vi "MGI Linear Fit.vi"(9 "Weights (equal)[]":dbl[](array[numeric]) format="%#.6g", 10 "Xin[]":dbl[](array[numeric]) format="%#.6g", 11 "Yin[]":dbl[](array[numeric]) format="%#.6g") -> (0 "Intercept":dbl, 1 "Slope":dbl, 2 "Xout[]":dbl[](array[numeric]), 3 "Yout[]":dbl[](array[numeric]))   [LabVIEW 2020]
doc: "Finds the least squares linear fit parameters for the provided data. If the range of x values is not greater than the range of y values, then the fit is performed with the x and y values reversed, with the outputs converted back to the original orientation. If the optional Weights input is empty or unwired, then the weights used in the fit are all set to 1 (equal weighting).\n\nAuthored by David A Moore\nsupport@mooregoodideas.com\nwww.mooregoodideas.com\n\nCopyright (c) 2010, Moore Good Ideas, Inc.\n\nAll rights reserved.\n\nRedistribution and use in source and binary forms, with or without modification, are permitted provided that the following conditions are met:\n\n * Redistributions of source code must retain the above copyright notice, this list of conditions and the following disclaimer.\n * Redistributions in binary form must reproduce the above copyright notice, this list of conditions and the following disclaimer in the documentation and/or other materials provided with the distribution.\n * Neither the name of Moore Good Ideas, Inc. nor the names of its contributors may be used to endorse or promote products derived from this software without specific prior written permission.\n\nTHIS SOFTWARE IS PROVIDED BY THE COPYRIGHT HOLDERS AND CONTRIBUTORS \"AS IS\" AND ANY EXPRESS OR IMPLIED WARRANTIES, INCLUDING, BUT NOT LIMITED TO, THE IMPLIED WARRANTIES OF MERCHANTABILITY AND FITNESS FOR A PARTICULAR PURPOSE ARE DISCLAIMED. IN NO EVENT SHALL THE COPYRIGHT OWNER OR CONTRIBUTORS BE LIABLE FOR ANY DIRECT, INDIRECT, INCIDENTAL, SPECIAL, EXEMPLARY, OR CONSEQUENTIAL DAMAGES (INCLUDING, BUT NOT LIMITED TO, PROCUREMENT OF SUBSTITUTE GOODS OR SERVICES; LOSS OF USE, DATA, OR PROFITS; OR BUSINESS INTERRUPTION) HOWEVER CAUSED AND ON ANY THEORY OF LIABILITY, WHETHER IN CONTRACT, STRICT LIABILITY, OR TORT (INCLUDING NEGLIGENCE OR OTHERWISE) ARISING IN ANY WAY OUT OF THE USE OF THIS SOFTWARE, EVEN IF ADVISED OF THE POSSIBILITY OF SUCH DAMAGE."
uses:
  <vilib>/Analysis/NI_AALPro.lvlib
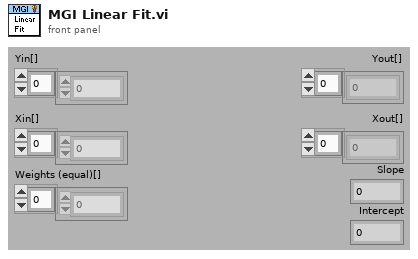
[diagram p1: front panel]
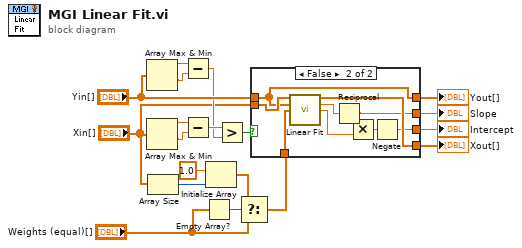
[diagram p0: block diagram]
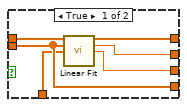
[diagram p2: hidden frame]
diagram:
  n1 = Array Max & Min(array="Yin[]") -> (max value=w16:dbl, min value=w17:dbl)  [unwired: 2 out]
  n2 = Array Max & Min(array="Xin[]") -> (max value=w19:dbl, min value=w18:dbl)  [unwired: 2 out]
  n3 = Array Size(array="Xin[]") -> (size(s)=w3:i32)
  n4 = Subtract(x=w16, y=w17) -> (x-y=w13:dbl)
  n5 = Subtract(x=w19, y=w18) -> (x-y=w14:dbl)
  n6 = Empty Array?(array="Weights (equal)[]") -> (empty?=w7:bool)
  n7 = Initialize Array(1.0 ("element"), w3) -> (w2:dbl[])
  n8 = Greater?(x=w14, y=w13) -> (0:w12:bool)
  n9 = Select(t=w2, s=w7, f="Weights (equal)[]") -> (s? t:f=w1:dbl[])
  n10 = case shown="False" w12 {
    tunnel: "Xin[]" -> [w21 w32]
    tunnel: "Yin[]" -> [w25 w31]
    tunnel: [w24 w31] -> w9
    tunnel: [w23 w29] -> w10
    tunnel: [w22 w27] -> w11
    tunnel: [w21 w33] -> w8
    tunnel: w1 -> [w20 w26]
    frame True {
      n11 = call <vilib>:"Linear Fit.vi"("Y"=w25, "X"=w21, "Weight"=w20) -> ("Best Linear Fit"=w24:dbl[], "slope"=w23:dbl, "intercept"=w22:dbl)  [unwired: 3 in, 7 out]
    }
    frame False {
      n12 = call <vilib>:"Linear Fit.vi"("Y"=w32, "X"=w31, "Weight"=w26) -> ("Best Linear Fit"=w33:dbl[], "slope"=w34:dbl, "intercept"=w28:dbl)  [unwired: 3 in, 7 out]
      n13 = Reciprocal(x=w34) -> (1/x=w29:dbl)
      n14 = Multiply(x=w29, y=w28) -> (x*y=w30:dbl)
      n15 = Negate(x=w30) -> (-x=w27:dbl)
    }
  }
  "Intercept" <- w11
  "Slope" <- w10
  "Yout[]" <- w9
  "Xout[]" <- w8
